vi "Ke2400 Measurement Current.vi"(8 "error in (no error)":errorcluster, 11 "VISA in":refnum<visa-resource-name>) -> (0 "error out":errorcluster, 2 "uA":string, 3 "VISA Out":refnum<visa-resource-name>)   [LabVIEW 2012]
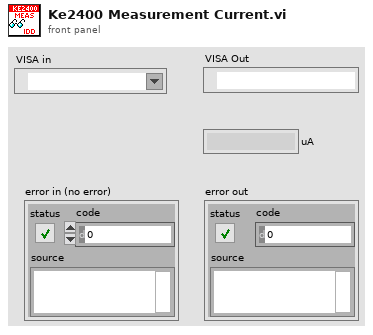
[diagram p1: front panel]
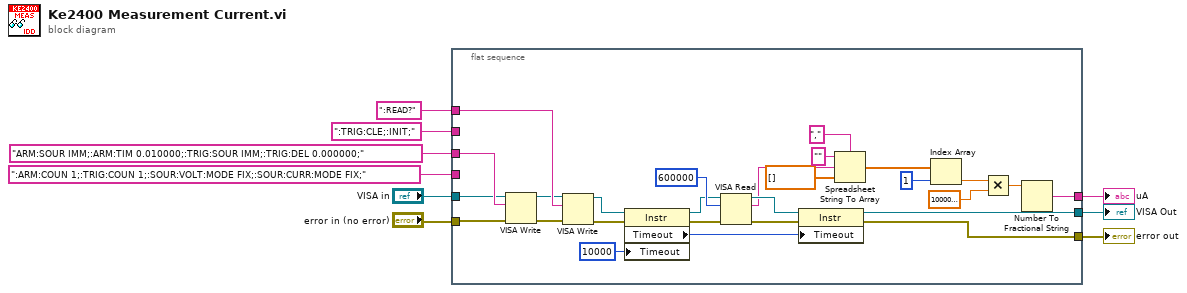
[diagram p0: block diagram]
diagram:
  n1 = flat-sequence {
    tunnel: [w21] -> w9
    tunnel: "VISA in" -> [w19]
    tunnel: "error in (no error)" -> [w18]
    tunnel: [w32] -> w6
    tunnel: [w24] -> w5
    tunnel: "ARM:SOUR IMM;:ARM:TIM 0.010000;:TRIG:SOUR IMM;:TRIG:DEL 0.000000;" ("resulting string") -> [w31]
    tunnel: ":TRIG:CLE;:INIT;" ("write buffer") -> [_]
    tunnel: ":READ?" ("write buffer") -> [w30]
    tunnel: ":ARM:COUN 1;:TRIG:COUN 1;:SOUR:VOLT:MODE FIX;:SOUR:CURR:MODE FIX;" ("write buffer") -> [_]
    frame #0 {
      n2 = VISA Write(VISA resource name=w19, write buffer=w31, error in (no error)=w18) -> (VISA resource name out=w17:refnum<visa-resource-name>, error out=w16:errorcluster)  [unwired: 1 out]
      n3 = VISA Write(VISA resource name=w17, write buffer=w30, error in (no error)=w16) -> (VISA resource name out=w28:refnum<visa-resource-name>, error out=w29:errorcluster)  [unwired: 1 out]
      n4 = property class="Instr"(reference=w28, error in=w29, "Timeout"=u32 10000 ("General Settings:Timeout Value")) -> (reference out=w27:refnum<visa-resource-name>, error out=w26:errorcluster, "Timeout"=w23:u32)
      n5 = VISA Read(VISA resource name=w27, byte count=u32 600000, error in (no error)=w26) -> (VISA resource name out=w25:refnum<visa-resource-name>, read buffer=w14:string, error out=w22:errorcluster)  [unwired: 1 out]
      n6 = property class="Instr"(reference=w25, error in=w22, "Timeout"=w23) -> (reference out=w24:refnum<visa-resource-name>, error out=w21:errorcluster)
      n7 = Spreadsheet String To Array(delimiter (Tab)=",", format string="", spreadsheet string=w14, array type (2D Dbl)=sgl[] []) -> (array=w10:sgl[])
      n8 = Index Array(array=w10, index=1) -> (element=w34:sgl)
      n9 = Multiply(x=w34, y=sgl 1000000.0) -> (x*y=w36:sgl)
      n10 = Number To Fractional String(number=w36) -> (F-format string=w32:string)  [unwired: 3 in]
    }
  }
  "error out" <- w9
  "uA" <- w6
  "VISA Out" <- w5
